vi "string to EIP channel.vi"(10 "channel data":string, 11 "identifier":string) -> (3 "channel in":refnum<class "EIP Tags Channel.lvclass">)   [LabVIEW 2013, in "EIP Tags Channel.lvclass"]
uses:
  EIP Tags Channel.lvclass
  <vilib>/NI/Tag Bus/tag/Data Type.ctl
  <vilib>/NI/Tag Bus Module Framework/channel/channel classification.ctl
  <vilib>/NI/Tag Bus/tag/tag descriptor.lvclass/tag descriptor.ctl
  <vilib>/NI/Tag Bus Module Framework/channel/TBM channel.lvclass/TBM channel.ctl
  EIP Tags Channel.lvclass/EIP Tags Channel.ctl
  <vilib>/NI/Tag Bus Module Framework/root configuration/TBM configuration.lvclass
  <vilib>/NI/Tag Bus/tag/tag descriptor.lvclass
  <vilib>/NI/Tag Bus Module Framework/channel/TBM channel.lvclass
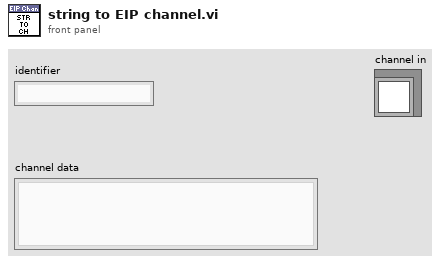
[diagram p1: front panel]
types:
  T1 = typedef "TBM channel.lvclass/channel classification.ctl" = enum16{"input data", "output data", "processing parameter", "processing result"}
  T2 = typedef "tag bus.lvlib/tag descriptor.lvclass/Data Type.ctl" = enum16{"Double", "Single", "I64", "I32", "I16", "I8", "U64", "U32", "U16", "U8", "Boolean", "String", "Array of Double", "Array of Single", "Array of I64", "Array of I32", "Array of I16", "Array of I8", "Array of U64", "Array of U32", "Array of U16", "Array of U8", "Array of Boolean", "Array of String"}
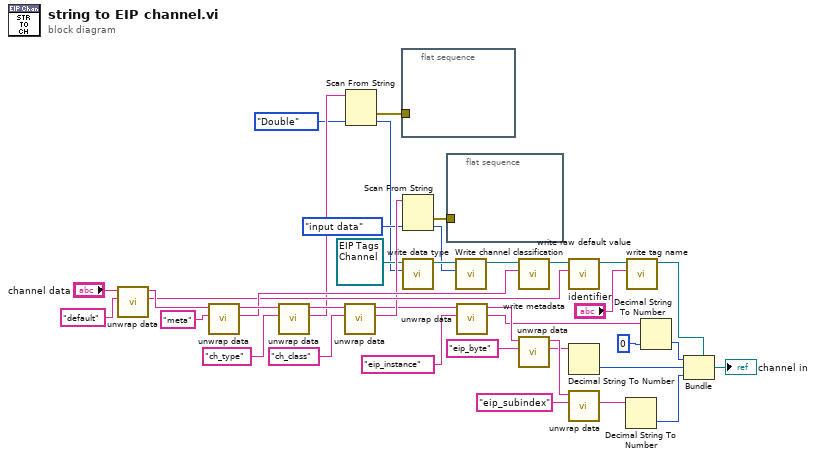
[diagram p0: block diagram]
diagram:
  n1 = call <vilib>:"unwrap data.vi"("identifier"="default", "data to unwrap"="channel data") -> ("unwrapped data"=w30:string, "remaining string"=w39:string)  [unwired: 8 in]
  n2 = call <vilib>:"unwrap data.vi"("identifier"="meta", "data to unwrap"=w39) -> ("unwrapped data"=w31:string, "remaining string"=w35:string)  [unwired: 8 in]
  n3 = call <vilib>:"unwrap data.vi"("identifier"="ch_type", "data to unwrap"=w35) -> ("unwrapped data"=w29:string, "remaining string"=w36:string)  [unwired: 8 in]
  n4 = call <vilib>:"unwrap data.vi"("identifier"="ch_class", "data to unwrap"=w36) -> ("unwrapped data"=w27:string, "remaining string"=w12:string)  [unwired: 8 in]
  n5 = Scan From String(input string=w29, default 1=Data_Type."Double" ("data type")) -> (error out=w25:errorcluster, output 1=w18:T2)  [unwired: 3 in, 2 out]
  n6 = flat-sequence {
    tunnel: w25 -> [_]
    frame #0 {
    }
  }
  n7 = Scan From String(input string=w27, default 1=channel_classification."input data" ("channel classification")) -> (error out=w24:errorcluster, output 1=w16:T1)  [unwired: 3 in, 2 out]
  n8 = call <vilib>:"write data type.vi"("data type"=w18, "system tag in"=refnum<class "EIP Tags Channel.lvclass"> refnum ("EthernetIP Channel.lvclass")) -> ("system tag out"=w19:refnum<class "EIP Tags Channel.lvclass">)  [unwired: 8 in, 1 out]
  n9 = flat-sequence {
    tunnel: w24 -> [_]
    frame #0 {
    }
  }
  n10 = call <vilib>:"Write channel classification.vi"("channel classification"=w16, "channel in"=w19) -> ("channel out"=w17:refnum<class "EIP Tags Channel.lvclass">)  [unwired: 8 in, 1 out]
  n11 = call <vilib>:"unwrap data.vi"("identifier"="eip_instance", "data to unwrap"=w12) -> ("unwrapped data"=w9:string, "remaining string"=w13:string)  [unwired: 8 in]
  n12 = call <vilib>:"write metadata.vi"("metadata"=w31, "system tag in"=w17) -> ("system tag out"=w32:refnum<class "EIP Tags Channel.lvclass">)  [unwired: 8 in, 1 out]
  n13 = call <vilib>:"unwrap data.vi"("identifier"="eip_byte", "data to unwrap"=w13) -> ("unwrapped data"=w8:string, "remaining string"=w10:string)  [unwired: 8 in]
  n14 = call <vilib>:"write raw default value.vi"("raw default"=w30, "system tag in"=w32) -> ("system tag out"=w20:refnum<class "EIP Tags Channel.lvclass">)  [unwired: 8 in, 1 out]
  n15 = Decimal String To Number(string=w8) -> (number=w5:i32)  [unwired: 2 in, 1 out]
  n16 = call <vilib>:"unwrap data.vi"("identifier"="eip_subindex", "data to unwrap"=w10) -> ("unwrapped data"=w7:string)  [unwired: 8 in, 1 out]
  n17 = Decimal String To Number(string=w7) -> (number=w6:i32)  [unwired: 2 in, 1 out]
  n18 = call <vilib>:"write tag name.vi"("name"="identifier", "system tag in"=w20) -> ("system tag out"=w2:refnum<class "EIP Tags Channel.lvclass">)  [unwired: 8 in, 1 out]
  n19 = Decimal String To Number(string=w9, default (0L)=u32 0 ("default (0 I32)")) -> (number=w3:u32)  [unwired: 1 in, 1 out]
  n20 = Bundle(cluster=w2, w3, w5, w6) -> (→"channel in":refnum<class "EIP Tags Channel.lvclass">)
